vi "SetRoomSides.vi"(8 "error in (no error)":errorcluster, 9 "Room":refnum<class "Room.lvclass">, 10 "RoomSides":T1[](array[typedef]), 11 "MazeGame in":refnum<class "MazeGame.lvclass">) -> (0 "error out":errorcluster, 3 "MazeGame out":refnum<class "MazeGame.lvclass">)   [LabVIEW 2020, in "FactoryMethod.lvlib" / "ParameterizedFactoryMethod.lvlib" / "MazeGame.lvclass"]
uses:
  MazeGame.lvclass
  NoParametrizedFactoryMethod/MazeGame/Private/TypeDef/RoomElement.ctl
  GoFcommonClasses/MazeSite/MazeSite.lvclass
  GoFcommonClasses/Direction.ctl
  GoFcommonClasses/ConcreteMazeSite/Room/Room.lvclass
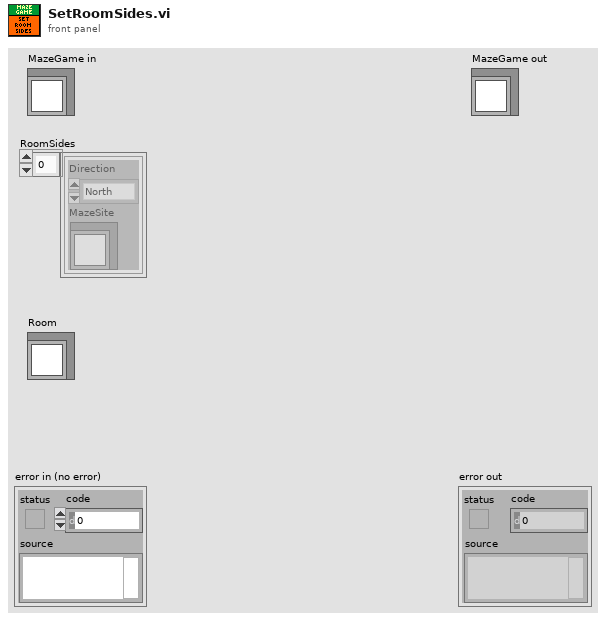
[diagram p1: front panel]
types:
  T1 = typedef "Room.lvclass/RoomElement.ctl" = cluster{"Direction":T2, "MazeSite":refnum<class "MazeSite.lvclass">}
  T2 = typedef "Direction.ctl" = enum32{"North", "South", "East", "West"}
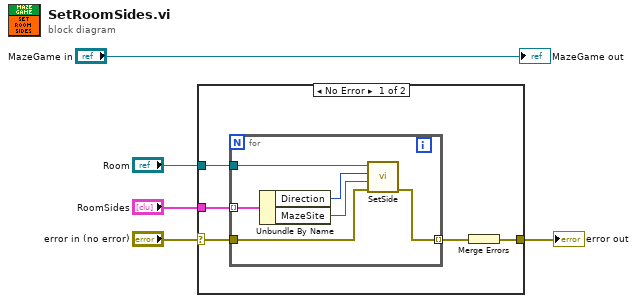
[diagram p0: block diagram]
diagram:
  n1 = case shown="No Error" "error in (no error)" {
    selector: "error in (no error)" -> [w8 w17]
    tunnel: [w6 w17] -> w4
    tunnel: "RoomSides" -> [w10 _]
    tunnel: "Room" -> [w9 _]
    frame No Error {
      n2 = for {
        tunnel: w10 -> [w15] mode=indexing
        tunnel: w9 -> [w16]
        tunnel: w8 -> [w12]
        tunnel: [w11] -> w7 mode=indexing
        n3 = Unbundle By Name(w15) -> ("Direction"=w14:T2, "MazeSite"=w13:refnum<class "MazeSite.lvclass">)
        n4 = call "SetSide.vi"("error in (no error)"=w12, "MazeSite"=w13, "Direction"=w14, "Room in"=w16) -> ("error out"=w11:errorcluster)  [unwired: 6 in, 1 out]
      }
      n5 = Merge Errors(w7) -> (w6:errorcluster)
    }
    frame Error {
    }
  }
  "error out" <- w4
  "MazeGame out" <- "MazeGame in"
